vi "replace_all_in_string.vi"(10 "replace_string":string, 11 "string_in":string) -> (3 "string_out":string)   [LabVIEW 2023, in "Error Handling Interface.lvlib" / "Error.lvclass"]
doc: "Replaces all special carachters \"~\" in the string with the replace_string input content"
uses:
  Error.lvclass
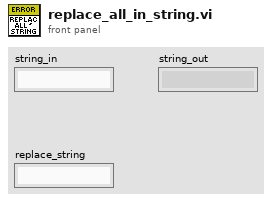
[diagram p1: front panel]
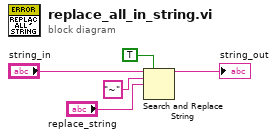
[diagram p0: block diagram]
diagram:
  n1 = Search and Replace String(replace all?=TRUE ("replace all? (F)"), input string="string_in", search string="~", replace string="replace_string") -> (result string=→"string_out":string)  [unwired: 4 in, 3 out]
